vi "Test Base64 Image Encoding.vi"() -> ()   [LabVIEW 2013]
panel:
  out "string out (base64-encoded)":string
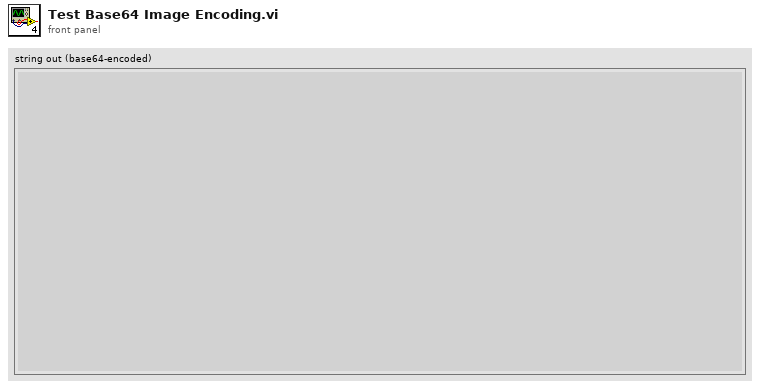
[diagram p1: front panel]
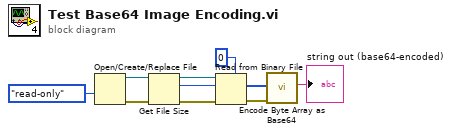
[diagram p0: block diagram]
diagram:
  n1 = Open/Create/Replace File(access (0:read/write)=enum16{"read/write", "read-only", "write-only"}."read-only") -> (refnum out=w7:refnum<file>, error out=w8:errorcluster)  [unwired: 5 in, 1 out]
  n2 = Get File Size(file=w7, error in=w8) -> (refnum out=w6:refnum<file>, size (in bytes)=w4:i64, 0:w5:errorcluster)
  n3 = Read from Binary File(5:u8 0, 8:w5, 10:w4, 11:w6) -> (0:w2:errorcluster, 2:w3:u8[])  [unwired: 2 in, 2 out]
  n4 = call "Encode Byte Array as Base64.vi"("error in (no error)"=w2, "unsigned byte array"=w3) -> ("string out (base64-encoded)"=→"string out (base64-encoded)":string)  [unwired: 8 in, 1 out]
